vi "Write Timestamp.vi"(8 "error in (no error)":errorcluster, 9 "Default If Not Found":timestamp, 10 "Name":string, 11 "IConfiguration in":refnum<class "IConfiguration.lvclass">) -> (0 "error out":errorcluster, 3 "IConfiguration out":refnum<class "IConfiguration.lvclass">)   [LabVIEW 2020, in "Configuration.lvlib" / "IConfiguration.lvclass"]
uses:
  <vilib>/gpm_packages/@cs/Configuration/Source/IConfiguration/IConfiguration.lvclass
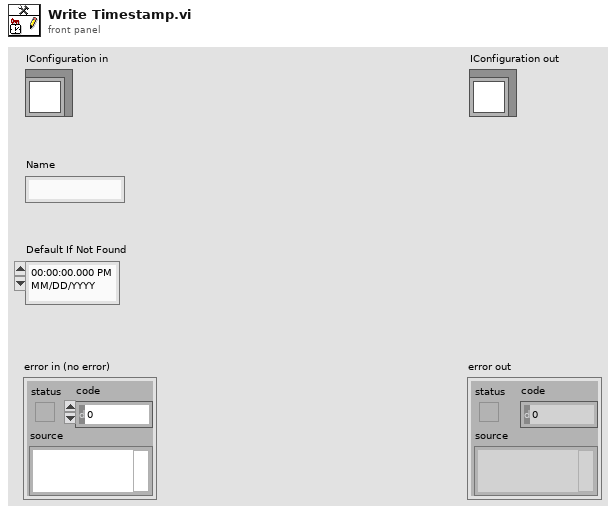
[diagram p1: front panel]
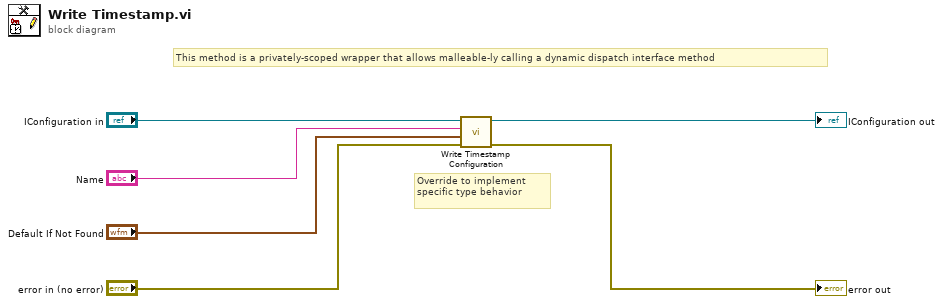
[diagram p0: block diagram]
diagram:
  # "Override to implement\nspecific type behavior"
  # "This method is a privately-scoped wrapper that allows malleable-ly calling a dynamic dispatch interface method"
  n1 = call-dynamic "Write Timestamp Configuration.vi"("error in (no error)"="error in (no error)", "Value"="Default If Not Found", "Name"="Name", "IConfiguration in"="IConfiguration in") -> ("error out"=→"error out":errorcluster, "IConfiguration out"=→"IConfiguration out":refnum<class "IConfiguration.lvclass">)  [unwired: 6 in]
